vi "E4_ExDiag.vi"() -> ()   [LabVIEW 2025]
panel:
  out "Numeric":i32
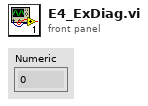
[diagram p1: front panel]
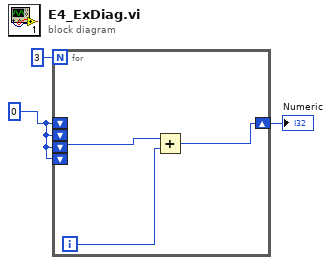
[diagram p0: block diagram]
diagram:
  w2 = 0
  n1 = for {
    N: 3 -> [_]
    shift-right: [w4] -> w1
    shift-left: w2 -> [_]
    shift-left: w2 -> [_]
    shift-left: w2 -> [_]
    shift-left: w2 -> [w5]
    i -> [w6]
    n2 = Add(x=w5, y=w6) -> (x+y=w4:i32)
  }
  "Numeric" <- w1
